vi "hot_plate_control_subVI.vi"(3 "Array":dbl[](array[numeric])) -> (0 "Numeric":dbl)   [LabVIEW 2021]
panel:
  out "Warmer\nON":bool
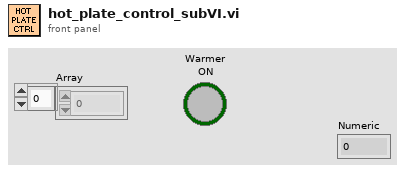
[diagram p1: front panel]
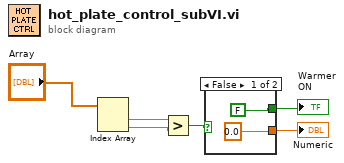
[diagram p0: block diagram]
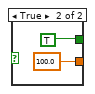
[diagram p2: hidden frame]
diagram:
  n1 = Index Array(array="Array") -> (element #1=w5:dbl, element #2=w4:dbl)  [unwired: 2 in]
  n2 = Greater?(x=w5, y=w4) -> (0:w3:bool)
  n3 = case shown="False" w3 {
    tunnel: [FALSE TRUE] -> w2
    tunnel: [0.0 100.0] -> w1
    frame False {
    }
    frame True {
    }
  }
  "Warmer\nON" <- w2
  "Numeric" <- w1
